vi "e.gate ASCII Read All Variables.vi"(8 "error in":errorcluster, 11 "e.gate Configuration in":T1 {"StartTime" format="%#.10f"; "dActTimeToSecondFactor" format="%#.10f"; "StartTimeToDayFactor" format="%#_10f"}) -> (0 "error IO":errorcluster, 2 "Array":dbl[](array[numeric]) caption="Variables", 3 "e.gate Configuration out":T1 {"StartTime" format="%#.10f"; "dActTimeToSecondFactor" format="%#.10f"; "StartTimeToDayFactor" format="%#_10f"})   [LabVIEW 2016]
doc: "<B>AMC - Analytik & Messtechnik GmbH Chemnitz</B>\n\nLabVIEW Drivers for e.gate / e.pac series from Gantner Instruments\n\nThis VI reads all defined values from a device specified by <B>connection ID In</B>."
uses:
  e.gate Configuration.ctl
  e.gate Channel Data.ctl
  e.gate Data Type.ctl
  e.gate Protocol Type.ctl
  e.gate Module  Data.ctl
  e.gateHSP_DLLhandle.ctl
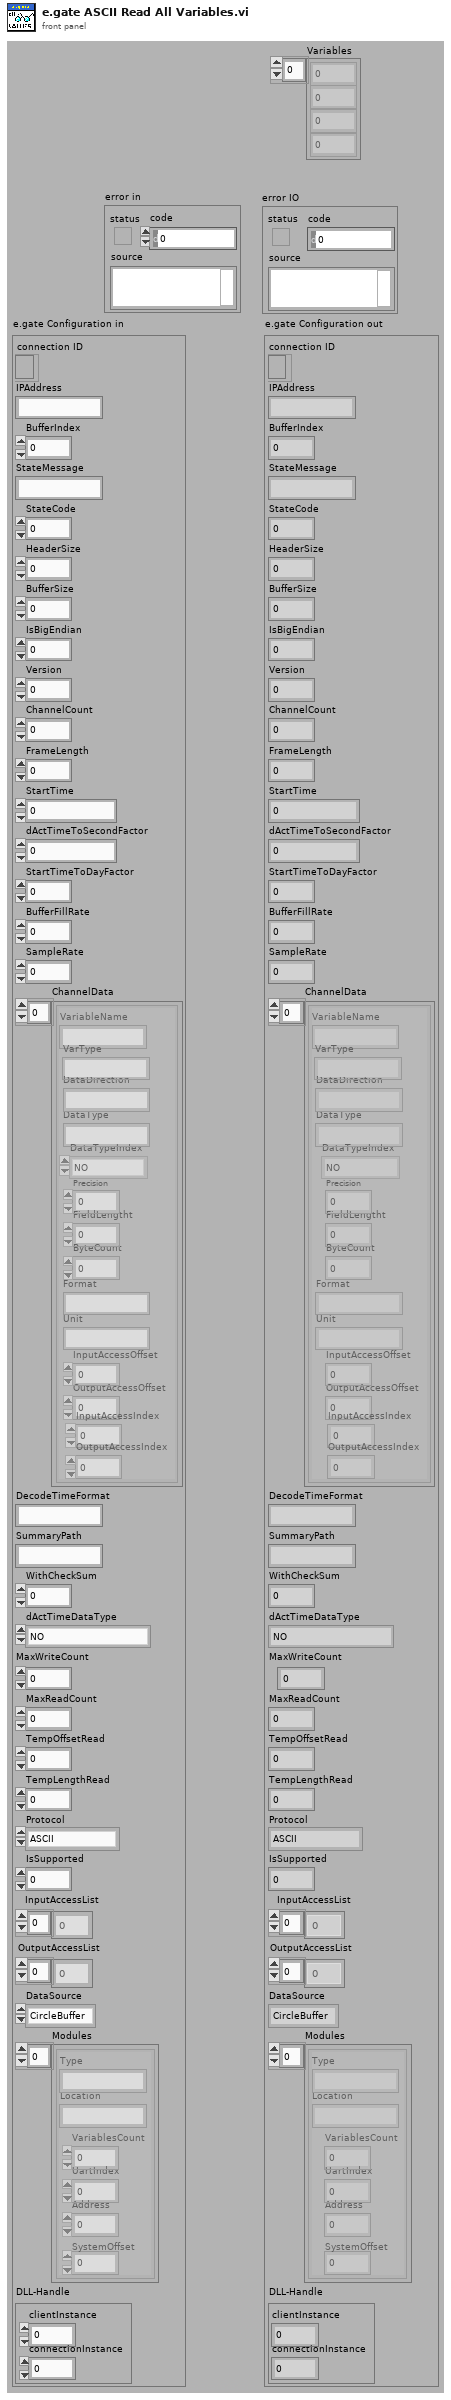
[diagram p1: front panel]
types:
  T1 = typedef "e.gate Configuration.ctl" = cluster{"connection ID":refnum<k5>, "IPAddress":string, "BufferIndex":i32, "StateMessage":string, "StateCode":i8, "HeaderSize":i32, "BufferSize":i32, "IsBigEndian":i32, "Version":i32, "ChannelCount":i32, "FrameLength":i32, "StartTime":dbl, "dActTimeToSecondFactor":dbl, "StartTimeToDayFactor":dbl, "BufferFillRate":dbl, "SampleRate":dbl, "ChannelData":T2[], "DecodeTimeFormat":string, "SummaryPath":string, "WithCheckSum":i32, "dActTimeDataType":T3, "MaxWriteCount":i32, "MaxReadCount":i32, "TempOffsetRead":i32, "TempLengthRead":i32, "Protocol":T4, "IsSupported":i32, "InputAccessList":i32[], "OutputAccessList":i32[], "DataSource":enum16{"CircleBuffer", "test.con Logger", "test.con Archive"}, "Modules":T5[], "DLL-Handle":T6}
  T2 = typedef "e.gate Channel Data.ctl" = cluster{"VariableName":string, "DataDirection":string, "DataType":string, "DataTypeIndex":T3, "Precision":i16, "FieldLengtht":i16, "ByteCount":i32, "Format":string, "Unit":string, "InputAccessOffset":i32, "OutputAccessOffset":i16, "InputAccessIndex":i16, "OutputAccessIndex":i16, "VarType":string}
  T3 = typedef "e.gate Data Type.ctl" = enum16{"NO", "BOOL", "SINT8", "USINT8", "SINT16", "USINT16", "SINT32", "USINT32", "FLOAT", "SET8", "SET16", "SET32", "DOUBLE", "SINT64", "USINT64", "SET64"}
  T4 = typedef "e.gate Protocol Type.ctl" = enum16{"ASCII", "HighspeedPort Online", "HighspeedPort Buffer", "eGateHighspeedPortDLL "}
  T5 = typedef "e.gate Module  Data.ctl" = cluster{"Type":string, "Location":string, "VariablesCount":i16, "UartIndex":i16, "Address":i16, "SystemOffset":i16}
  T6 = typedef "e.gateHSP_DLLhandle.ctl" = cluster{"clientInstance":i32, "connectionInstance":i32}
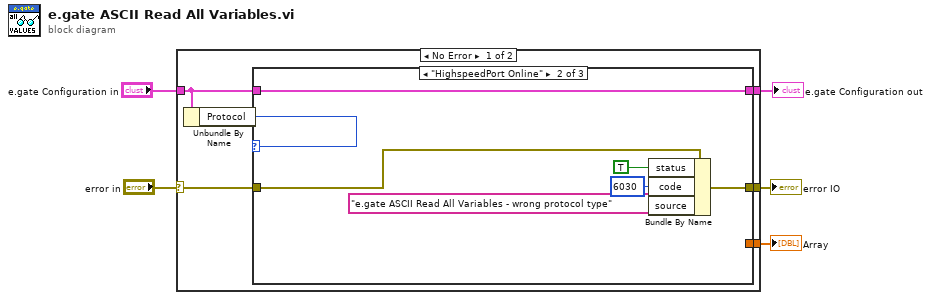
[diagram p0: block diagram]
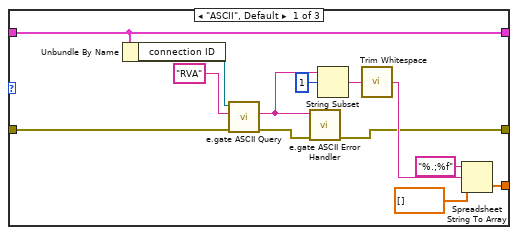
[diagram p2: hidden frame]
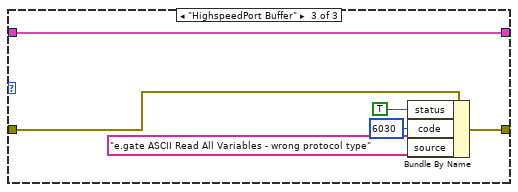
[diagram p3: hidden frame]
diagram:
  n1 = case shown="No Error" "error in" {
    selector: "error in" -> [w10 w38]
    tunnel: [w9 w38] -> w4
    tunnel: [w11 _] -> w5
    tunnel: "e.gate Configuration in" -> [w7 w37]
    tunnel: [w6 w37] -> w1
    frame No Error {
      n2 = Unbundle By Name(w7) -> ("Protocol"=w8:T4)
      n3 = case shown="\"HighspeedPort Online\"" w8 {
        tunnel: [w20 _ _] -> w11
        tunnel: w10 -> [w13 w29 w32]
        tunnel: [w18 w28 w33] -> w9
        tunnel: w7 -> [w12 w30 w31]
        tunnel: [w12 w30 w31] -> w6
        frame "ASCII", Default {
          n4 = Unbundle By Name(w12) -> ("connection ID"=w15:refnum<k5>)
          n5 = call "e.gate ASCII Query.vi"("error in (no error)"=w13, "Command"="RVA" ("format string"), "connection ID In"=w15) -> ("error out"=w17:errorcluster, "Response"=w16:string)  [unwired: 6 in, 1 out]
          n6 = call "e.gate ASCII Error Handler.vi"("error in (no error)"=w17, "String"=w16) -> ("error out"=w18:errorcluster)  [unwired: 9 in]
          n7 = String Subset(string=w16, offset (0)=1) -> (substring=w23:string)  [unwired: 1 in]
          n8 = call <vilib>:"Trim Whitespace.vi"("string"=w23) -> ("trimmed string"=w22:string)  [unwired: 1 in]
          n9 = Spreadsheet String To Array(format string="%.;%f", spreadsheet string=w22, array type (2D Dbl)=dbl[] []) -> (array=w20:dbl[])  [unwired: 1 in]
        }
        frame "HighspeedPort Online" {
          n10 = Bundle By Name(cluster=w29, "status"=TRUE, "code"=6030, "source"="e.gate ASCII Read All Variables - wrong protocol type") -> (w28:errorcluster)
        }
        frame "HighspeedPort Buffer" {
          n11 = Bundle By Name(cluster=w32, "status"=TRUE, "code"=6030, "source"="e.gate ASCII Read All Variables - wrong protocol type") -> (w33:errorcluster)
        }
      }
    }
    frame Error {
    }
  }
  "Array" <- w5
  "error IO" <- w4
  "e.gate Configuration out" <- w1
